vi "Check Objective settings validity.vi"(10 "Default Calibration":T1, 11 "Loaded \nCalibration Config":T1) -> (3 "Loaded \nCalibration Config":T1)   [LabVIEW 2020]
uses:
  Typedefs/Calibration config.ctl
  Typedefs/Objective Config.ctl
  Typedefs/Prechirper Cal Config.ctl
  Typedefs/PreChirper constants.ctl
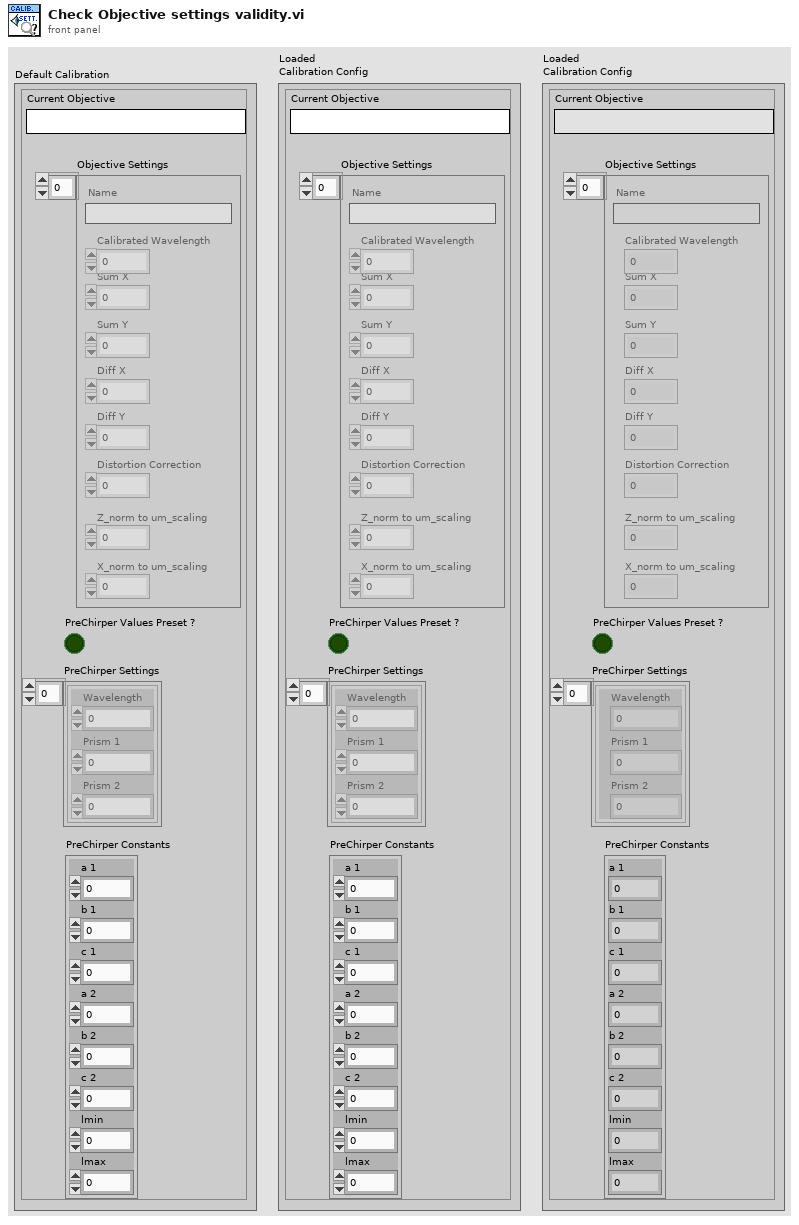
[diagram p1: front panel]
types:
  T1 = typedef "Calibration config.ctl" = cluster{"Current Objective":string, "Objective Settings":T2[], "PreChirper Values Preset ?":bool, "PreChirper Settings":T3[], "PreChirper Constants":T4}
  T2 = typedef "Objective Config.ctl" = cluster{"Name":string, "Sum X":dbl, "Sum Y":dbl, "Diff X":dbl, "Diff Y":dbl, "Distortion Correction":dbl, "Z_norm to um_scaling":dbl, "X_norm to um_scaling":dbl, "Calibrated Wavelength":dbl}
  T3 = typedef "Prechirper Cal Config.ctl" = cluster{"Wavelength":i32, "Prism 1":i32, "Prism 2":i32}
  T4 = typedef "PreChirper constants.ctl" = cluster{"a 1":i32, "b 1":i32, "c 1":i32, "a 2":i32, "b 2":i32, "c 2":i32, "lmin":i32, "lmax":i32}
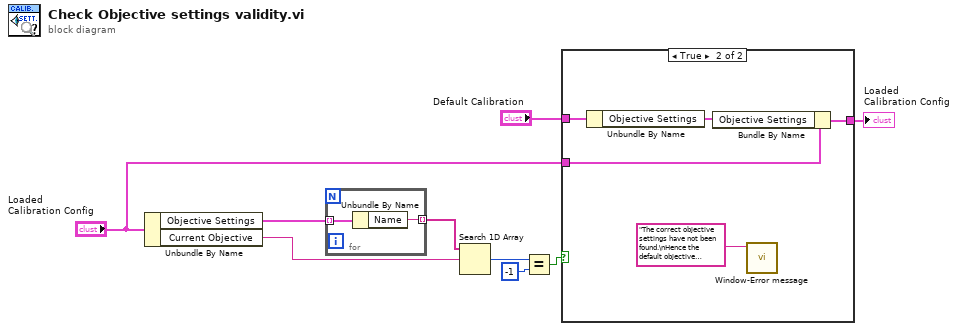
[diagram p0: block diagram]
diagram:
  n1 = Unbundle By Name("Loaded \nCalibration Config") -> ("Objective Settings"=w3:T2[], "Current Objective"=w5:string)
  n2 = for {
    tunnel: w3 -> [w11] mode=indexing
    tunnel: [w10] -> w4 mode=indexing
    n3 = Unbundle By Name(w11) -> ("Name"=w10:string)
  }
  n4 = Search 1D Array(1D array=w4, element=w5) -> (index of element=w6:i32)  [unwired: 1 in]
  n5 = Equal?(x=w6, y=-1) -> (x = y?=w8:bool)
  n6 = case shown="True" w8 {
    tunnel: "Default Calibration" -> [_ w17]
    tunnel: "Loaded \nCalibration Config" -> [w12 w16]
    tunnel: [w12 w14] -> w1
    frame False {
    }
    frame True {
      n7 = Unbundle By Name(w17) -> ("Objective Settings"=w15:T2[])
      n8 = Bundle By Name(cluster=w16, "Objective Settings"=w15) -> (w14:T1)
      n9 = call "Window-Error message.vi"("Message"="The correct objective settings have not been found.\nHence the default objective settings have been re-instated.\nPlease check the Calibration.ini file !") -> ()  [unwired: 10 in, 1 out]
    }
  }
  "Loaded \nCalibration Config" <- w1
